vi "define.vi"(8 "error in (no error)":errorcluster, 11 "TrajectoryAK101022Resonance in":refnum<class "TrajectoryAK101022Resonance.lvclass">) -> (0 "error out":errorcluster, 3 "TrajectoryAK101022Resonance out":refnum<class "TrajectoryAK101022Resonance.lvclass">)   [LabVIEW 2010, in "TrajectoryAK101022Resonance.lvclass"]
doc: "modal dialog on which the user can set the trajectory parameters"
uses:
  TrajectoryAK101022Resonance.lvclass
  filter_type_enum.ctl
  TrajectoryAK101022Resonance.lvclass/TrajectoryAK101022Resonance.ctl
panel:
  in  "Vy min(V)":dbl
  in  "Vy max(V)":dbl
  in  "Vz min(V)":dbl
  in  "Vz max(V)":dbl
  out "frame rate":dbl[unit]
  out "resonance frequency":dbl[unit]
  out "Number of z points":i32
  out "repetitions (volumes)":i32
  out "number of planes":i32
  out "step size":dbl[unit]
  out "z signal":dbl[unit][][](graph)
  in  "Filter on?":bool
  in  "z-Function type":enum32{"Sine", "tooth", "Stack", "Step"}(tab)=enum."tooth"
  out "ETL frequency":dbl[unit]=1.0 min=1.0
  in  "ETL amplitude conversion":dbl[unit]=12600.0
  in  "ETL phase delay":dbl[unit]=0.008726646259971648
  in  "angle fraction":dbl=1.0
  out "Lines per z step (sine)":i32=1 caption="lines per z step" min=1
  out "ETL frequency 2":dbl[unit]=1.0 caption="ETL frequency" min=1.0
  in  "ETL amplitude conversion 2":dbl[unit]=12600.0
  in  "ETL phase delay 2":dbl[unit]=0.008726646259971648
  in  "bi-directional? 2":bool
  in  "angle fraction 2":dbl=1.0
  out "Lines per z step (sine) 2":i32=1 caption="lines per z step" min=1
  in  "Level High (Step)":dbl caption="Level High"
  in  "Lines per z step (Step)":i32 caption="Lines per z step" min=1
  in  "Level overshoot (Step)":dbl caption="Level overshoot"
  in  "Level undershoot (Step)":dbl caption="Level undershoot"
  in  "Sample level high (Step)":u16 caption="Sample level high"
  in  "Sample overshoot (Step)":u16 caption="Sample overshoot"
  in  "Sample ramp (Step)":u16 caption="Sample ramp"
  in  "Sample undershoot (Step)":u16 caption="Sample undershoot"
  in  "filter type":T1
  in  "filter order":u16=2
  in  "low cutoff freq":dbl=0.125
  in  "high cutoff freq":dbl=0.45
  in  "button:cancel":bool
  in  "button:ok":bool
  # "Define TrajectoryAK101022Resonance"
  # "X galvo"
  # "Y galvo"
  # "Filtering"
  # "In this mode, the z signal is sine function."
  # "In this mode, the z signal is a tooth function."
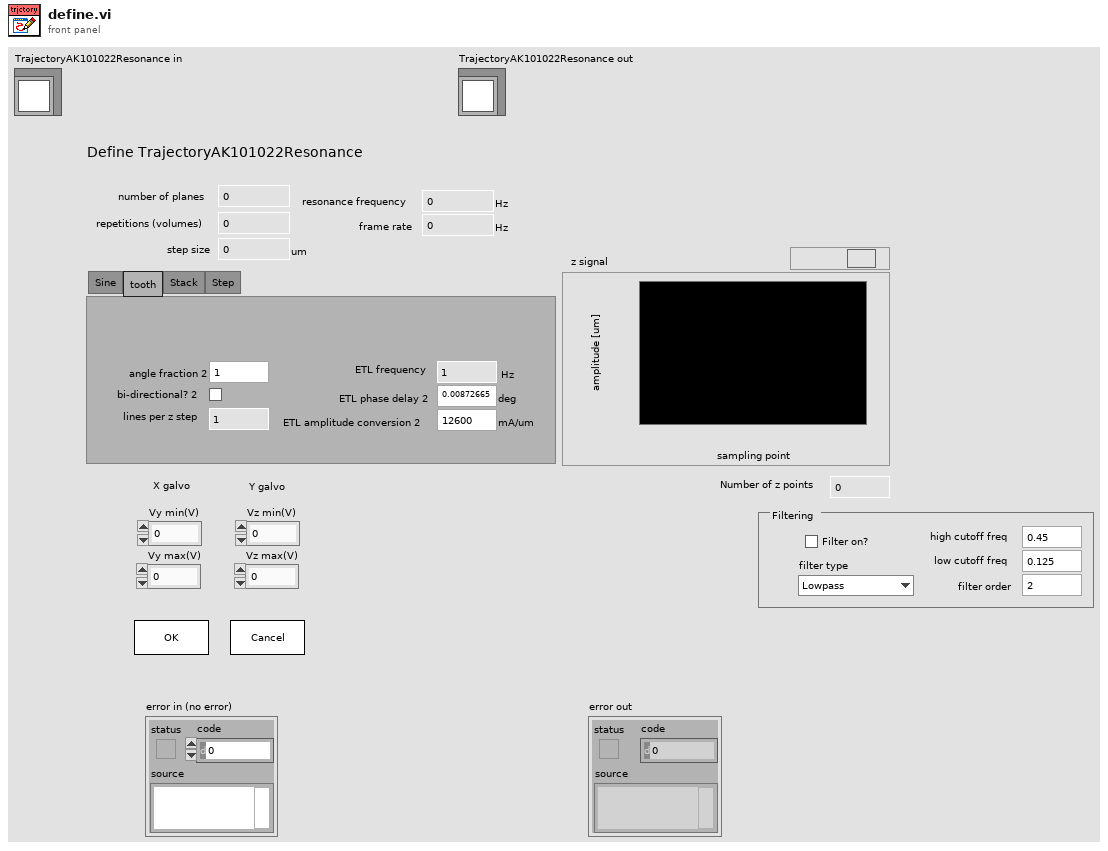
[diagram p1: front panel]
types:
  T1 = typedef "TrajectoryAK101022Resonance.lvclass/filter_type_enum.ctl" = enum16{"Lowpass", "Highpass", "Bandpass", "Bandstop"}
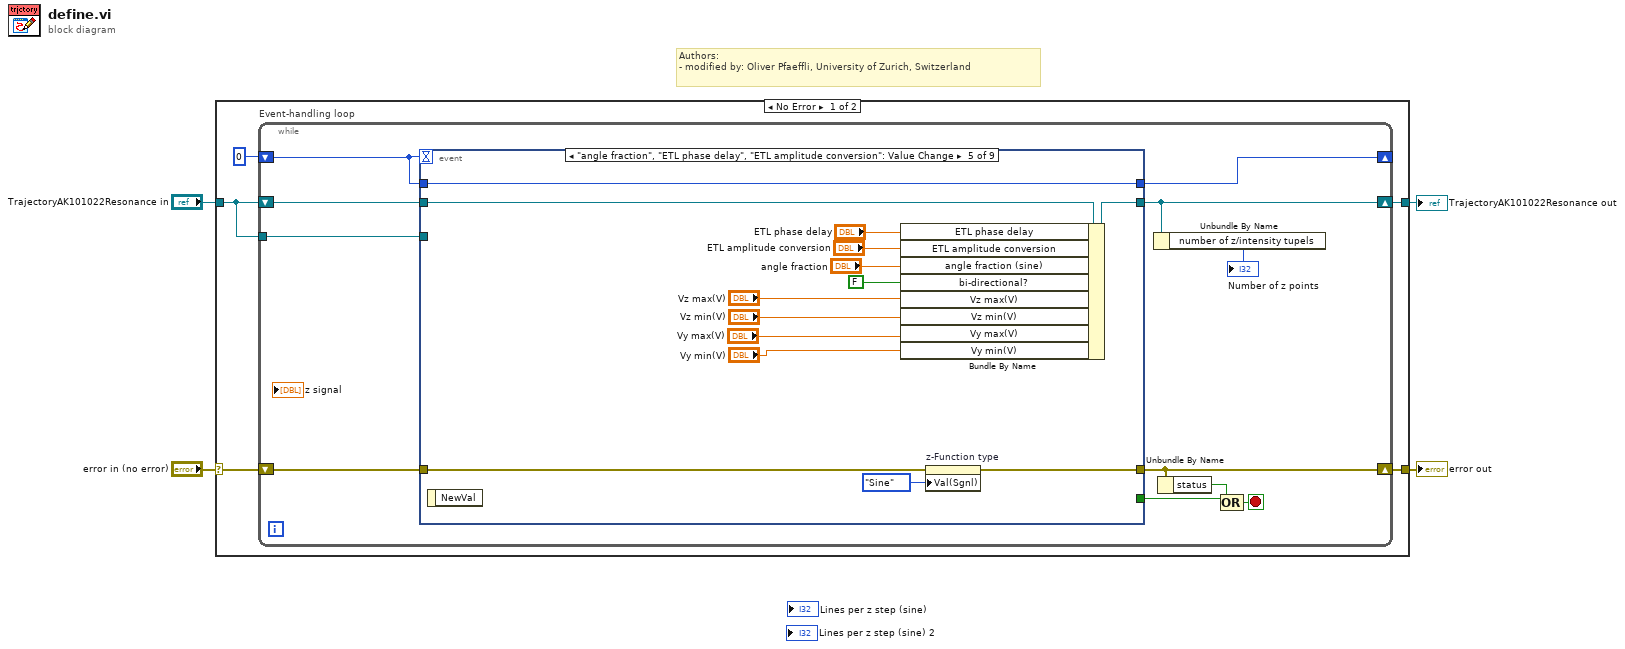
[diagram p0: block diagram]
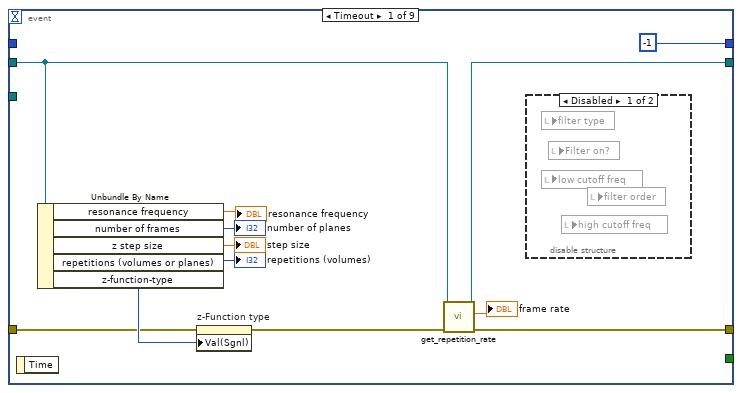
[diagram p2: hidden frame]
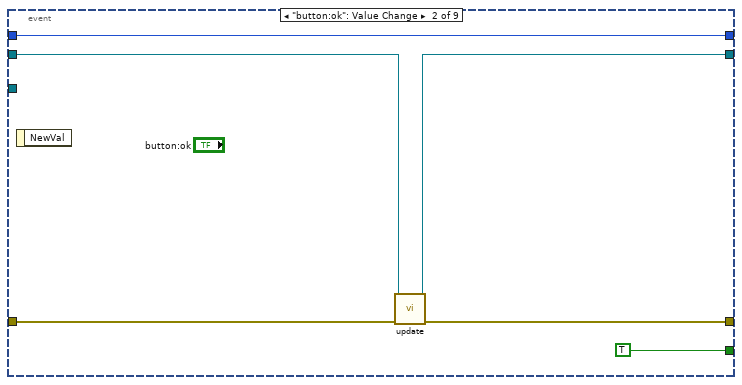
[diagram p4: hidden frame]
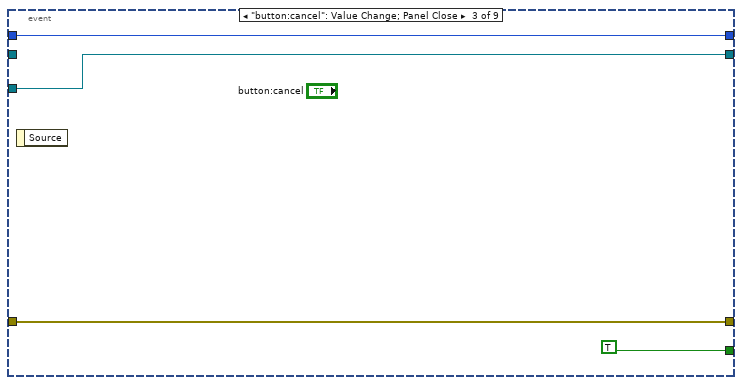
[diagram p5: hidden frame]
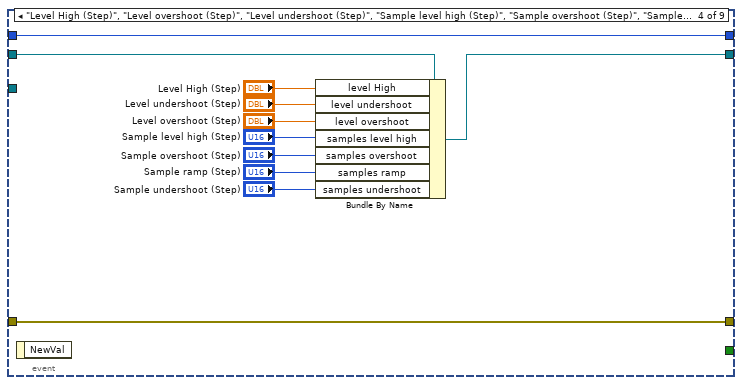
[diagram p6: hidden frame]
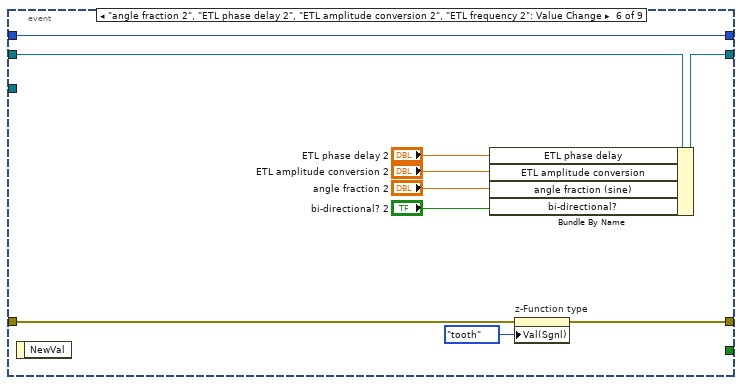
[diagram p7: hidden frame]
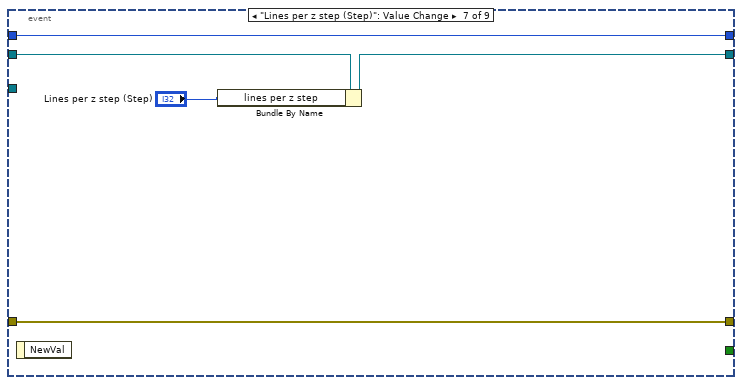
[diagram p8: hidden frame]
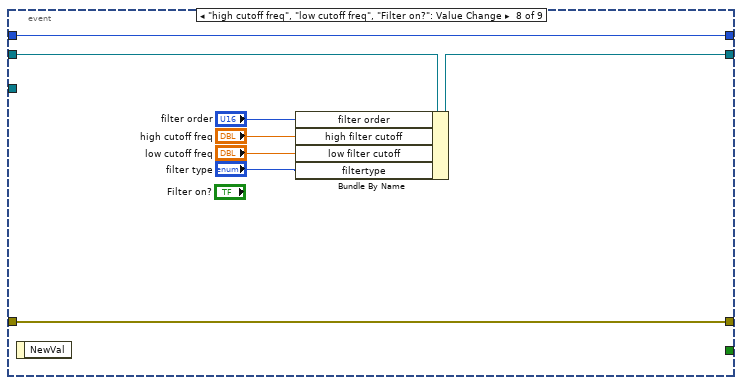
[diagram p9: hidden frame]
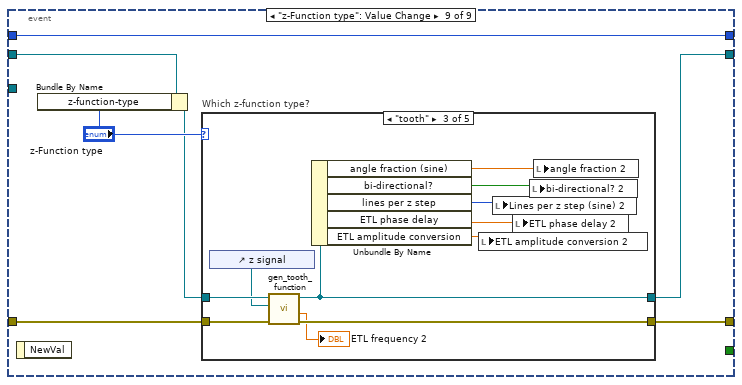
[diagram p10: hidden frame]
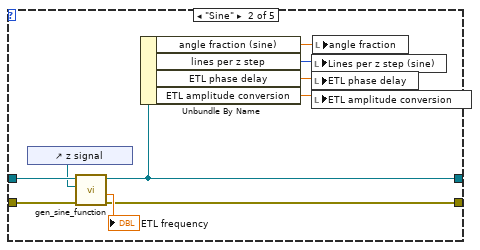
[diagram p12: hidden frame]
diagram:
  # "Authors: \n- modified by: Oliver Pfaeffli, University of Zurich, Switzerland"
  n1 = case shown="No Error" "error in (no error)" {
    selector: "error in (no error)" -> [w9 w126]
    tunnel: [w8 w126] -> w3
    tunnel: "TrajectoryAK101022Resonance in" -> [w5 w125]
    tunnel: [w7 w125] -> w1
    frame No Error {
      n2 = while "Event-handling loop" {
        shift-right: [w13] -> w8
        shift-left: w9 -> [w14]
        shift-right: [w16] -> _
        shift-left: 0 -> [w17]
        shift-right: [w11] -> w7
        shift-left: w5 -> [w18]
        tunnel: w5 -> [w15]
        stop <- w19 stop-if-true
        n3 = event shown="[4] \"angle fraction\", \"ETL phase delay\", \"ETL amplitude conversion\": Value Change" {
          selector: _ -> [_ _ _ _ _ _ _ _ _]
          dyn-events: _ -> [_ _ _ _ _ _ _ _ _]
          timeout: w17 -> [_ _ _ _ _ _ _ _ _]
          tunnel: w18 -> [w24 w33 _ w52 w60 w73 w81 w89 w97]
          tunnel: w17 -> [_ w38 w42 w43 w67 w77 w78 w83 w91]
          tunnel: [-1 w38 w42 w43 w67 w77 w78 w83 w91] -> w16
          tunnel: [w27 w36 w41 w51 w66 w76 w80 w88 w92] -> w11
          tunnel: w15 -> [_ _ w41 _ _ _ _ _ _]
          tunnel: w14 -> [w22 w34 w40 w53 w61 w74 w82 w90 w96]
          tunnel: [w26 w35 w40 w53 w62 w75 w82 w90 w95] -> w13
          tunnel: [_ TRUE TRUE _ _ _ _ _ _] -> w12
          event Timeout {
            n4 = event-data() -> ()  [unwired: 1 in, 1 out]
            n5 = Unbundle By Name(w24) -> ("resonance frequency"=→"resonance frequency":dbl[unit], "number of frames"=→"number of planes":i32, "z step size"=→"step size":dbl[unit], "repetitions (volumes or planes)"=→"repetitions (volumes)":i32, "z-function-type"=w23:enum16{"Sine", "tooth", "Stack", "Step"})
            n6 = property on="z-Function type" class="TabCtl (strict)"(error in=w22, "Val(Sgnl)"=w23) -> (error out=w21:errorcluster)  [unwired: 1 in, 1 out]
            n7 = call-dynamic "get_repetition_rate.vi"("error in (no error)"=w21, "GenericTrajectory in"=w24) -> ("error out"=w26:errorcluster, "repetition rate"=→"frame rate":dbl[unit], "GenericTrajectory out"=w27:refnum<class "TrajectoryAK101022Resonance.lvclass">)  [unwired: 7 in]
            n8 = disable-structure shown="Disabled" {
              frame Disabled {
                n9 = local read "filter type"() -> ()  [unwired: 1 in]
                n10 = local read "low cutoff freq"() -> ()  [unwired: 1 in]
                n11 = local read "Filter on?"() -> ()  [unwired: 1 in]
                n12 = local read "high cutoff freq"() -> ()  [unwired: 1 in]
                n13 = local read "filter order"() -> ()  [unwired: 1 in]
              }
              frame Enabled {
              }
            }
          }
          event "button:ok": Value Change {
            n14 = event-data() -> ()  [unwired: 1 in, 1 out]
            n15 = call-dynamic "update.vi"("error in (no error)"=w34, "TrajectoryAK101022Resonance in"=w33) -> ("error out"=w35:errorcluster, "TrajectoryAK101022Resonance out"=w36:refnum<class "TrajectoryAK101022Resonance.lvclass">)  [unwired: 8 in]
          }
          event "button:cancel": Value Change; Panel Close {
            n16 = event-data() -> ()  [unwired: 1 in, 1 out]
          }
          event "Level High (Step)", "Level overshoot (Step)", "Level undershoot (Step)", "Sample level high (Step)", "Sample overshoot (Step)", "Sample ramp (Step)", "Sample undershoot (Step)": Value Change {
            n17 = event-data() -> ()  [unwired: 1 in, 1 out]
            n18 = Bundle By Name(cluster=w52, "level High"="Level High (Step)", "level undershoot"="Level undershoot (Step)", "level overshoot"="Level overshoot (Step)", "samples level high"="Sample level high (Step)", "samples overshoot"="Sample overshoot (Step)", "samples ramp"="Sample ramp (Step)", "samples undershoot"="Sample undershoot (Step)") -> (w51:refnum<class "TrajectoryAK101022Resonance.lvclass">)
          }
          event "angle fraction", "ETL phase delay", "ETL amplitude conversion": Value Change {
            n19 = event-data() -> ()  [unwired: 1 in, 1 out]
            n20 = Bundle By Name(cluster=w60, "ETL phase delay"="ETL phase delay", "ETL amplitude conversion"="ETL amplitude conversion", "angle fraction (sine)"="angle fraction", "bi-directional?"=FALSE ("settings.bi-directional?"), "Vz max(V)"="Vz max(V)", "Vz min(V)"="Vz min(V)", "Vy max(V)"="Vy max(V)", "Vy min(V)"="Vy min(V)") -> (w66:refnum<class "TrajectoryAK101022Resonance.lvclass">)
            n21 = property on="z-Function type" class="TabCtl (strict)"(error in=w61, "Val(Sgnl)"=enum32{"Sine", "tooth", "Stack", "Step"}."Sine" ("Value (Signaling)")) -> (error out=w62:errorcluster)  [unwired: 1 in, 1 out]
          }
          event "angle fraction 2", "ETL phase delay 2", "ETL amplitude conversion 2", "ETL frequency 2": Value Change {
            n22 = event-data() -> ()  [unwired: 1 in, 1 out]
            n23 = Bundle By Name(cluster=w73, "ETL phase delay"="ETL phase delay 2", "ETL amplitude conversion"="ETL amplitude conversion 2", "angle fraction (sine)"="angle fraction 2", "bi-directional?"="bi-directional? 2") -> (w76:refnum<class "TrajectoryAK101022Resonance.lvclass">)
            n24 = property on="z-Function type" class="TabCtl (strict)"(error in=w74, "Val(Sgnl)"=enum32{"Sine", "tooth", "Stack", "Step"}."tooth" ("Value (Signaling)")) -> (error out=w75:errorcluster)  [unwired: 1 in, 1 out]
          }
          event "Lines per z step (Step)": Value Change {
            n25 = event-data() -> ()  [unwired: 1 in, 1 out]
            n26 = Bundle By Name(cluster=w81, "lines per z step"="Lines per z step (Step)") -> (w80:refnum<class "TrajectoryAK101022Resonance.lvclass">)
          }
          event "high cutoff freq", "low cutoff freq", "Filter on?": Value Change {
            n27 = event-data() -> ()  [unwired: 1 in, 1 out]
            n28 = Bundle By Name(cluster=w89, "filter order"="filter order", "high filter cutoff"="high cutoff freq", "low filter cutoff"="low cutoff freq", "filtertype"="filter type") -> (w88:refnum<class "TrajectoryAK101022Resonance.lvclass">)
          }
          event "z-Function type": Value Change {
            n29 = event-data() -> ()  [unwired: 1 in, 1 out]
            n30 = Bundle By Name(cluster=w97, "z-function-type"="z-Function type") -> (w93:refnum<class "TrajectoryAK101022Resonance.lvclass">)
            n31 = case "Which z-function type?" shown="\"tooth\"" "z-Function type" {
              tunnel: w96 -> [w99 w108 w119 w122 w124]
              tunnel: [w99 w107 w118 w122 w124] -> w95
              tunnel: w93 -> [w98 w106 w120 w121 w123]
              tunnel: [w98 w104 w115 w121 w123] -> w92
              frame Default {
              }
              frame "Sine" {
                n32 = control-ref of="z signal"() -> (w100:refnum<vi>)
                n33 = call "gen_sine_function.vi"("error in (no error)"=w108, "z signal graph ref"=w100, "TrajectoryAK101022Resonance in"=w106) -> ("error out"=w107:errorcluster, "z-frequency"=→"ETL frequency":dbl[unit], "TrajectoryAK101022Resonance out"=w104:refnum<class "TrajectoryAK101022Resonance.lvclass">)  [unwired: 5 in, 1 out]
                n34 = Unbundle By Name(w104) -> ("angle fraction (sine)"=w105:dbl, "lines per z step"=w103:i32, "ETL phase delay"=w102:dbl[unit], "ETL amplitude conversion"=w101:dbl[unit])
                n35 = local write "Lines per z step (sine)"(w103) -> ()
                n36 = local write "ETL phase delay"(w102) -> ()
                n37 = local write "ETL amplitude conversion"(w101) -> ()
                n38 = local write "angle fraction"(w105) -> ()
              }
              frame "tooth" {
                n39 = control-ref of="z signal"() -> (w116:refnum<vi>)
                n40 = call "gen_tooth_function.vi"("error in (no error)"=w119, "z signal graph ref"=w116, "TrajectoryAK101022Resonance in"=w120) -> ("error out"=w118:errorcluster, "z-frequency"=→"ETL frequency 2":dbl[unit], "TrajectoryAK101022Resonance out"=w115:refnum<class "TrajectoryAK101022Resonance.lvclass">)  [unwired: 5 in, 1 out]
                n41 = Unbundle By Name(w115) -> ("angle fraction (sine)"=w114:dbl, "bi-directional?"=w113:bool, "lines per z step"=w112:i32, "ETL phase delay"=w111:dbl[unit], "ETL amplitude conversion"=w110:dbl[unit])
                n42 = local write "ETL amplitude conversion 2"(w110) -> ()
                n43 = local write "Lines per z step (sine) 2"(w112) -> ()
                n44 = local write "ETL phase delay 2"(w111) -> ()
                n45 = local write "bi-directional? 2"(w113) -> ()
                n46 = local write "angle fraction 2"(w114) -> ()
              }
              frame "Stack" {
              }
              frame "Step" {
              }
            }
          }
        }
        n47 = Unbundle By Name(w11) -> ("number of z/intensity tupels"=→"Number of z points":i32)
        n48 = Unbundle By Name(w13) -> ("status"=w20:bool)
        n49 = Compound Arithmetic op=OR(w20, w12) -> (w19:bool)
      }
    }
    frame Error {
    }
  }
  "error out" <- w3
  "TrajectoryAK101022Resonance out" <- w1
